vi "AuMT8852B Request EUT Name on Connect.vi"(5 "Enabled? (F)":bool, 7 "Set/Get (Set)":enum16{"Set", "Get"}(ring), 8 "error in (no error)":errorcluster, 10 "Script (3)":i32=3, 11 "VISA session":refnum<visa-resource-name>) -> (0 "error out":errorcluster, 2 "error code":i32, 3 "VISA session out":refnum<visa-resource-name>, 4 "Enabled? out":bool)   [LabVIEW 2017]
doc: "Anritsu MT8852B Bluetooth Tester\n\nWhen a test or script is run, the MT8850 will first make a connection to the EUT. During this connection process the EUT features and user friendly name are normally requested. This command allows the request for the user friendly name not to be requested as part of this connection sequence.\n\nINPUTS\nSet/Get - whether the value is being sent to or retrieved from the instrument.\nEnabled? - whether or not the MT8850 will request the EUT name when a connection is established.\n\nOUTPUTS\nEnabled? out - whether or not the MT8850 is currently set to request the EUT name when a connection is established."
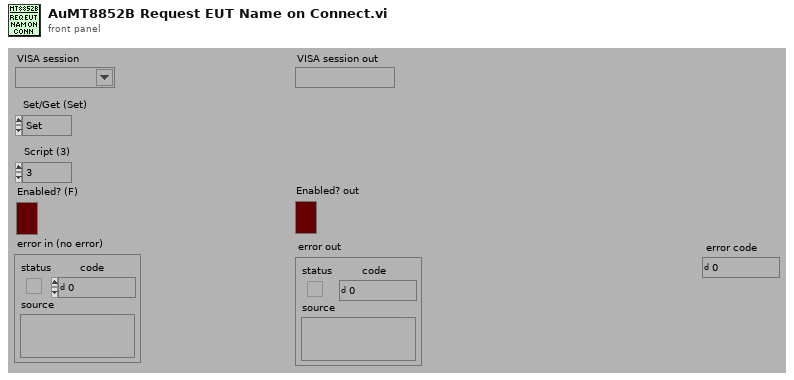
[diagram p1: front panel]
types:
  T1 = enum16{"Simulate", "Range check", "Cache", "Query instrument status"}
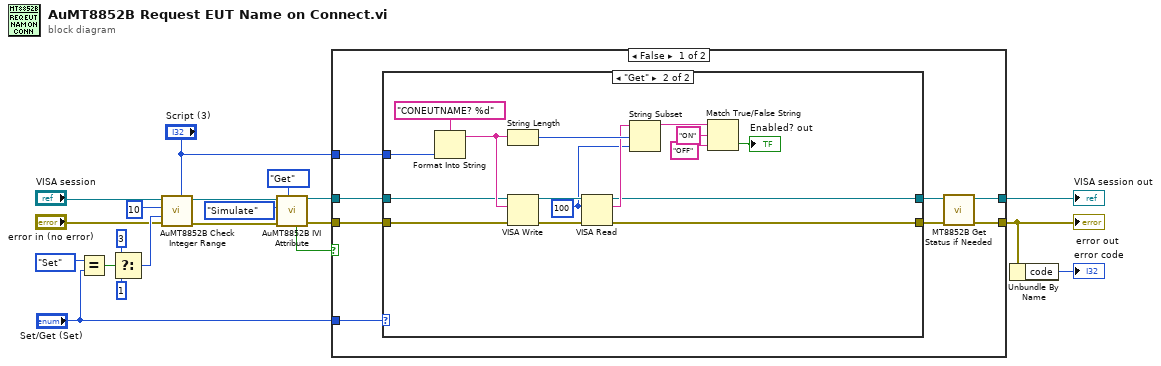
[diagram p0: block diagram]
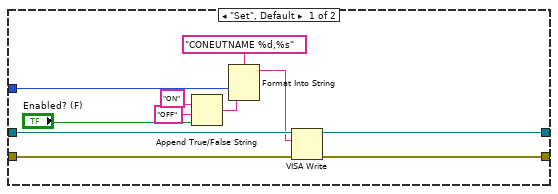
[diagram p2: hidden frame]
diagram:
  n1 = Equal?(x=enum16{"Set", "Get"}."Set" ("y"), y="Set/Get (Set)") -> (x = y?=w12:bool)
  n2 = Select(t=3, s=w12, f=1) -> (s? t:f=w9:i32)
  n3 = call <instrlib>:"AuMT8852B Check Integer Range.vi"("Value (0)"="Script (3)", "error in (no error)"="error in (no error)", "Lower limit (-1)"=w9, "Upper limit (1)"=10, "VISA session"="VISA session") -> ("error out"=w6:errorcluster, "VISA session out"=w7:refnum<visa-resource-name>)  [unwired: 5 in]
  n4 = call <instrlib>:"AuMT8852B IVI Attribute.vi"("Set/Get (Set)"=enum16{"Set", "Get"}."Get", "error in (no error)"=w6, "Flag (Simulate)"=T1."Simulate", "VISA session"=w7) -> ("error out"=w16:errorcluster, "VISA session out"=w17:refnum<visa-resource-name>, "Value out"=w15:bool)  [unwired: 5 in]
  n5 = case shown="False" w15 {
    tunnel: [w25 w56] -> w20
    tunnel: [w24 w57] -> w13
    tunnel: w17 -> [w28 w56]
    tunnel: w16 -> [w27 w57]
    tunnel: "Script (3)" -> [w22 _]
    tunnel: "Set/Get (Set)" -> [w21 _]
    frame False {
      n6 = case shown="\"Get\"" w21 {
        tunnel: w28 -> [w39 w49]
        tunnel: w27 -> [w38 w48]
        tunnel: [w37 w47] -> w26
        tunnel: [w36 w46] -> w23
        tunnel: w22 -> [w33 w45]
        frame "Set", Default {
          n7 = Append True/False String(1:"Enabled? (F)", 2:"OFF" ("false string"), 3:"ON" ("true string")) -> (0:w29:string)  [unwired: 1 in]
          n8 = Format Into String(format string="CONEUTNAME %d,%s" ("Format String"), w33, w29) -> (resulting string=w34:string)  [unwired: 2 in, 1 out]
          n9 = VISA Write(VISA resource name=w39, write buffer=w34, error in (no error)=w38) -> (VISA resource name out=w37:refnum<visa-resource-name>, error out=w36:errorcluster)  [unwired: 1 out]
        }
        frame "Get" {
          w44 = u32 100 ("byte count (0)")
          n10 = Format Into String(format string="CONEUTNAME? %d" ("Format String"), w45) -> (resulting string=w52:string)  [unwired: 2 in, 1 out]
          n11 = String Length(string=w52) -> (length=w51:i32)
          n12 = VISA Write(VISA resource name=w49, write buffer=w52, error in (no error)=w48) -> (VISA resource name out=w55:refnum<visa-resource-name>, error out=w54:errorcluster)  [unwired: 1 out]
          n13 = VISA Read(VISA resource name=w55, byte count=w44, error in (no error)=w54) -> (VISA resource name out=w47:refnum<visa-resource-name>, read buffer=w50:string, error out=w46:errorcluster)  [unwired: 1 out]
          n14 = String Subset(string=w50, offset (0)=w51, length (rest)=w44) -> (substring=w41:string)
          n15 = Match True/False String(2:"OFF" ("false string"), 3:"ON" ("true string"), 4:w41) -> (0:→"Enabled? out":bool)  [unwired: 1 out]
        }
      }
      n16 = call <instrlib>:"MT8852B Get Status if Needed.vi"("error in (no error)"=w23, "VISA session"=w26) -> ("error out"=w24:errorcluster, "VISA session out"=w25:refnum<visa-resource-name>)  [unwired: 8 in]
    }
    frame True {
    }
  }
  "VISA session out" <- w20
  "error out" <- w13
  n17 = Unbundle By Name(w13) -> ("code"=→"error code":i32)
